vi "Register Test.vi"(11 "Properties.Test in":refnum<class "Properties.Test.lvclass">) -> (3 "Properties.Test out":refnum<class "Properties.Test.lvclass">)   [LabVIEW 2013, in "Caraya.lvlib" / "Properties.Test.lvclass"]
uses:
  Properties.Test.lvclass
  Test Manager Message Test/Test-Data -- cluster.ctl
  Properties/Properties.lvclass/Properties.ctl
  Properties/Properties.lvclass
  Test Manager Message Test/TestManagerMsg.Test.lvclass
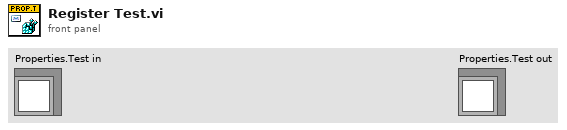
[diagram p1: front panel]
types:
  T1 = typedef "Caraya.lvlib/TestManagerMsg.Test.lvclass/Test-Data -- cluster.ctl" = cluster{"test-name":string, "call-chain":string[], "timestamp":timestamp}
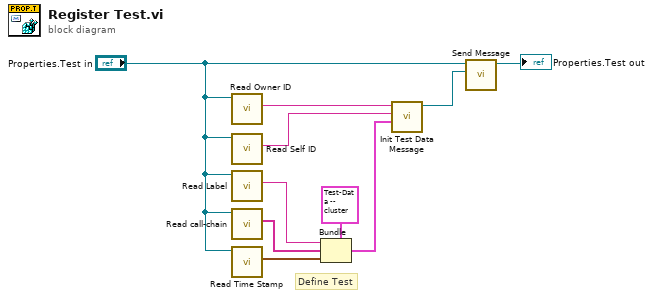
[diagram p0: block diagram]
diagram:
  # "Define Test"
  n1 = call "Read Owner ID.vi"("Properties in"="Properties.Test in") -> ("owner-id"=w2:string)  [unwired: 9 in, 1 out]
  n2 = call "Read Self ID.vi"("Properties in"="Properties.Test in") -> ("self-id"=w3:string)  [unwired: 9 in, 1 out]
  n3 = call "Read Label.vi"("Properties in"="Properties.Test in") -> ("Test Label"=w6:string)  [unwired: 9 in, 1 out]
  n4 = call "Read call-chain.vi"("Properties in"="Properties.Test in") -> ("call-chain"=w8:string[])  [unwired: 9 in, 1 out]
  n5 = call "Read Time Stamp.vi"("Properties in"="Properties.Test in") -> ("Time Stamp"=w7:timestamp)  [unwired: 9 in, 1 out]
  n6 = Bundle(cluster=T1 {"test-name"="", "call-chain"=[], "timestamp"=timestamp(3763321070.9484735 s since 1904-01-01)} ("Test Data"), "test-name"=w6, "call-chain"=w8, "timestamp"=w7) -> (w4:T1)
  n7 = call "Init Test Data Message.vi"("Test Data"=w4, "TestID"=w3, "CallerID"=w2) -> ("Message"=w9:refnum<class "TestManagerMsg.lvclass">)  [unwired: 8 in]
  n8 = call "Send Message.vi"("TestManagerMsg"=w9, "Properties in"="Properties.Test in") -> ("Properties out"=→"Properties.Test out":refnum<class "Properties.Test.lvclass">)  [unwired: 8 in, 1 out]
